vi "ADstar on a Dynamic Occupancy Grid - Copy.vi"() -> ()   [LabVIEW 2012]
doc: "This example continually replans a path from Start to Goal while following the best known path, including through obstacles if necessary.\nThe Anytime D* search algorithm is useful when the world or the robot's understanding of the world is changing. Anytime D* maintains more information than the A* search algorithm so the robot can backtrack and find a new path more easily if it discovers the original path will not work."
uses:
  <vilib>/robotics/Navigation/shared/WorldMap/OccupancyGridWorldMap/NI_Robotics_OccupancyGridWorldMap.lvclass
  <vilib>/robotics/Navigation/Anytime D Star/NI_Robotics_AnytimeDStar.lvclass
panel:
  in  "Step Through":bool
  in  "goal y":i32=49
  in  "goal x":i32=49
  out "Open List Size":i32(graph)=1665
  out "path on obstacles":dbl[][](graph)
  out "AD* Open Nodes":i32=1665 caption="size"
  out "Path Cost":dbl(graph)
  in  "Epsilon":i32=2 min=1
  out "AD* Path Cost":dbl caption="path cost"
  in  "y start":i32
  in  "x start":i32
  in  "Move Robot":i32=1 min=0
  in  "Overhaul":i32=25
  in  "step button":bool
  out "AD* Time":u32=117 caption="seconds"
  out "Compute Path Time":u32(graph)=117
  in  "stop":bool
  # "The Anytime D* search algorithm is useful when the world or the robot's understanding of the world is changing.  Anytime D* maintains more information\n than the A* search algorithm so the robot can backtrack and find a new path more easily if it discovers the original path will not work."
  # "This example continually replans a path from Start to Goal while \nfollowing the best known path, including through obstacles if necessary."
  # "Configuration"
  # "X"
  # "Y"
  # "Start"
  # "Goal"
  # "Run Mode"
  # "Run-time Control"
  # "Detection radius of robot's sensors."
  # "Number of steps the robot takes after each plan."
  # "Number of steps before AD* plans from scratch."
  # "1) Choose the Start and Goal location and the % Random Obstacles.\n2) Run the VI.\n3) Adjust the controls in the Run-time Controls section to see the \n     effect each option has on path planning\n4) Change the Run Mode to Single Step to pause after each time\n the AD* VI runs"
  # "A higher epsilon results in a faster but less optimal search."
  # "Continuous"
  # "Single Step"
  # "Robot"
  # "Obstacle"
  # "Unknown"
  # "Free"
  # "Path"
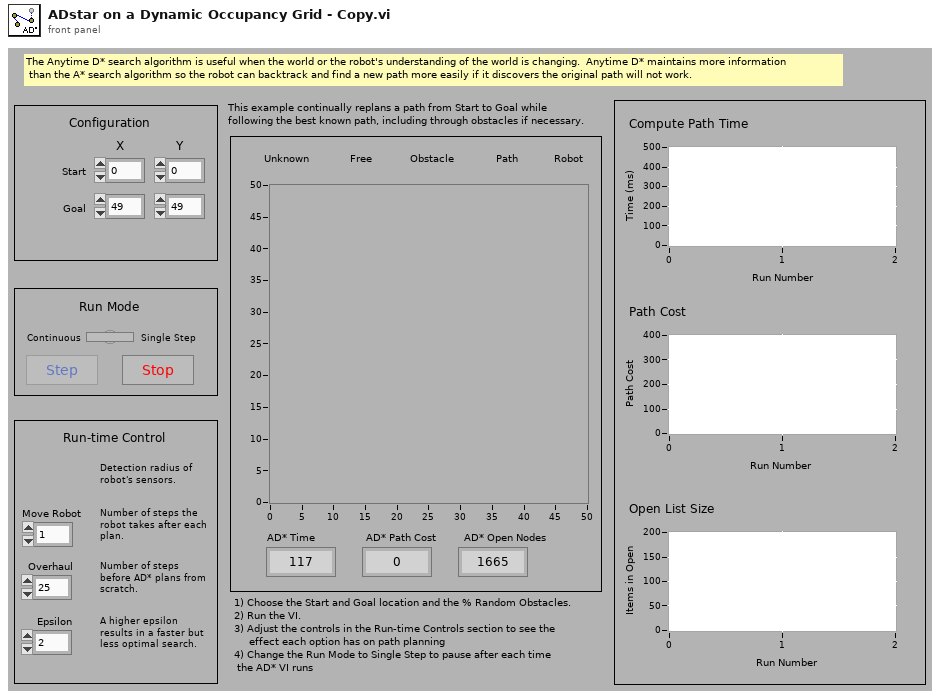
[diagram p1: front panel]
types:
  T1 = enum8{"Enabled", "Disabled", "Disabled and Grayed Out"}
  T2 = cluster{"epsilon":dbl, "run number":i32, "open list size":i32}
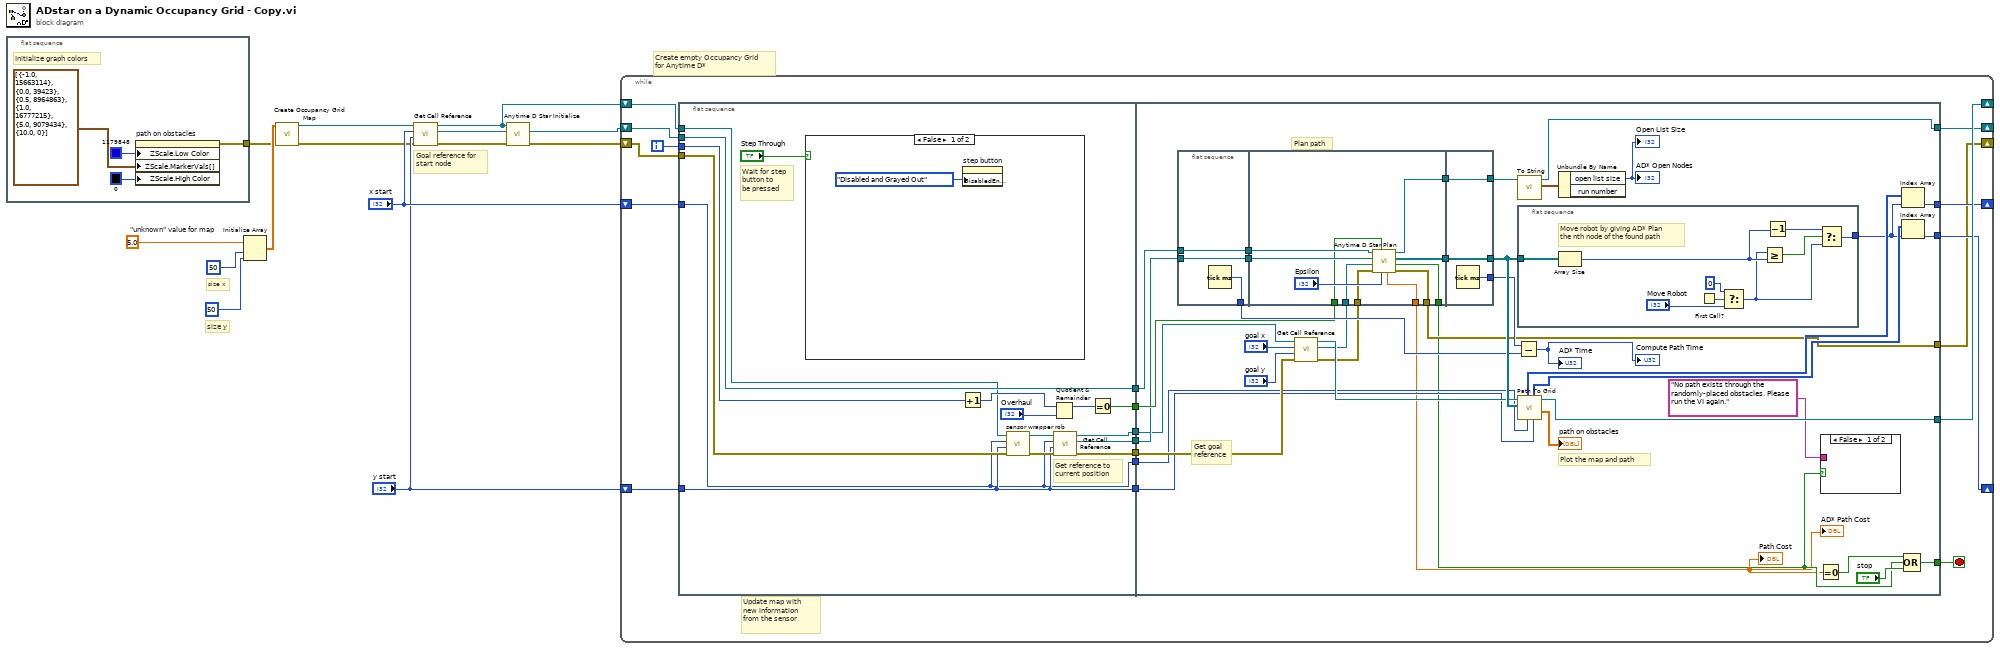
[diagram p0: block diagram]
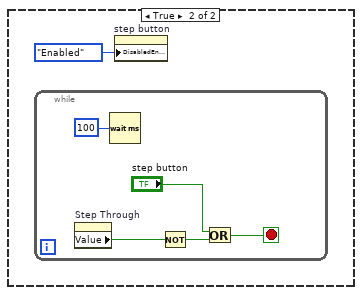
[diagram p2: hidden frame]
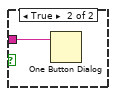
[diagram p3: hidden frame]
diagram:
  w12 = 5.0  # "unknown" value for map
  # "Goal reference for\nstart node"
  # "size y"
  # "size x"
  # "Create empty Occupancy Grid\nfor Anytime D*"
  n1 = flat-sequence {
    tunnel: [w15] -> w5
    frame #0 {
      # "Initialize graph colors"
      n2 = property on="path on obstacles" class="IntGraph (strict)"("ZScale.Low Color"=u32 1179848, "ZScale.MarkerVals[]"=cluster{dbl, u32}[] [{-1.0, 15663114}, {0.0, 39423}, {0.5, 8964863}, {1.0, 16777215}, {5.0, 9079434}, {10.0, 0}], "ZScale.High Color"=u32 0) -> (error out=w15:errorcluster)  [unwired: 2 in, 1 out]
    }
  }
  n3 = Initialize Array(w12, 50 ("y"), 50 ("x")) -> (w9:dbl[][])
  n4 = call <vilib>:"Create Occupancy Grid Map.vi"("error in (no error)"=w5, "occupancy grid"=w9) -> ("error out"=w7:errorcluster, "map reference out"=w2:refnum<data-value>)  [unwired: 8 in]
  n5 = call <vilib>:"Get Cell Reference.vi"("error in (no error)"=w7, "y"="y start", "x"="x start", "map reference in"=w2) -> ("error out"=w6:errorcluster, "cell reference"=w8:refnum<data-value>, "map reference out"=w3:refnum<data-value>)  [unwired: 4 in, 1 out]
  n6 = call <vilib>:"Anytime D Star Initialize.vi"("error in (no error)"=w6, "start reference"=w8, "map reference in"=w3) -> ("error out"=w1:errorcluster, "Anytime D*"=w4:refnum<class "NI_Robotics_AnytimeDStar.lvclass">)  [unwired: 7 in]
  n7 = while {
    shift-right: [w32] -> _
    shift-left: w4 -> [w37]
    shift-right: [w36] -> _
    shift-left: w3 -> [w22]
    shift-right: [w31] -> _
    shift-left: "x start" -> [w19]
    shift-right: [w30] -> _
    shift-left: "y start" -> [w20]
    shift-right: [w26] -> _
    shift-left: w1 -> [w21]
    i -> [w29]
    stop <- w23 stop-if-true
    # "Update map with new information\nfrom the sensor"
    n8 = flat-sequence {
      tunnel: w29 -> [w46]
      tunnel: w22 -> [w43]
      tunnel: w37 -> [w53]
      tunnel: [w53] -> w35
      tunnel: [w52] -> w34
      tunnel: [w51] -> w33
      tunnel: w19 -> [w38]
      tunnel: w20 -> [w39]
      tunnel: [w45] -> w28
      tunnel: w21 -> [w40]
      tunnel: [w44] -> w27
      tunnel: [w38] -> w25
      tunnel: [w39] -> w24
      tunnel: [w63] -> w23
      tunnel: [w97] -> w32
      tunnel: [w85] -> w36
      tunnel: [w78] -> w31
      tunnel: [w77] -> w30
      tunnel: w28 -> [w83]
      tunnel: w33 -> [w82]
      tunnel: w34 -> [w76]
      tunnel: w35 -> [w93]
      tunnel: w27 -> [w73]
      tunnel: [w69] -> w26
      tunnel: w25 -> [w68]
      tunnel: w24 -> [w67]
      frame #0 {
        # "Get reference to \ncurrent position"
        # "Wait for step\nbutton to\nbe pressed"
        n9 = case shown="False" "Step Through" {
          frame False {
            n10 = property on="step button" class="Bool"("DisabledEnum"=T1."Disabled and Grayed Out" ("Disabled")) -> ()  [unwired: 2 in, 2 out]
          }
          frame True {
            n11 = while {
              stop <- w58 stop-if-true
              n12 = property on="Step Through" class="Bool (strict)"() -> ("Value"=w56:bool)  [unwired: 2 in, 2 out]
              n13 = Wait (ms)(milliseconds to wait=u32 100) -> ()  [unwired: 1 out]
              n14 = Not(x=w56) -> (.not. x?=w57:bool)
              n15 = Or(x="step button", y=w57) -> (x .or. y?=w58:bool)
            }
            n16 = property on="step button" class="Bool"("DisabledEnum"=T1."Enabled" ("Disabled")) -> ()  [unwired: 2 in, 2 out]
          }
        }
        n17 = Increment(x=w46) -> (x+1=w48:i32)
        n18 = call "sensor wrapper rob.vi"("error in (no error)"=w40, "sensor y"=w39, "Sensor x"=w38, "map reference in"=w43) -> ("error out"=w41:errorcluster, "map reference out 2"=w42:refnum<data-value>)  [unwired: 6 in]
        n19 = Quotient & Remainder(x=w48, y="Overhaul") -> (x-y*floor(x/y)=w47:i32)  [unwired: 1 out]
        n20 = call <vilib>:"Get Cell Reference.vi"("error in (no error)"=w41, "y"=w39, "x"=w38, "map reference in"=w42) -> ("error out"=w44:errorcluster, "cell reference"=w51:refnum<data-value>, "map reference out"=w52:refnum<data-value>)  [unwired: 4 in, 1 out]
        n21 = Equal To 0?(x=w47) -> (x = 0?=w45:bool)
      }
      frame #1 {
        # "Plot the map and path"
        # "Get goal \nreference"
        # "Plan path"
        n22 = flat-sequence {
          tunnel: w93 -> [w110]
          tunnel: w82 -> [w111]
          tunnel: [w111] -> w92
          tunnel: [w110] -> w91
          tunnel: [w109] -> w87
          tunnel: [w118] -> w64
          tunnel: [w117] -> w62
          tunnel: w92 -> [w121]
          tunnel: w91 -> [w122]
          tunnel: [w119] -> w90
          tunnel: [w120] -> w89
          tunnel: w83 -> [w115]
          tunnel: w71 -> [w114]
          tunnel: w70 -> [w113]
          tunnel: [w112] -> w69
          tunnel: [w124] -> w96
          tunnel: [w125] -> w98
          tunnel: w90 -> [w125]
          tunnel: w89 -> [w124]
          tunnel: [w123] -> w88
          frame #0 {
            n23 = Tick Count (ms)() -> (millisecond timer value=w109:u32)
          }
          frame #1 {
            n24 = call <vilib>:"Anytime D Star Plan.vi"("epsilon"="Epsilon", "overhaul (F)"=w115, "error in (no error)"=w113, "new goal reference"=w114, "current reference"=w121, "Anytime D* in"=w122) -> ("error out"=w112:errorcluster, "no valid path exists"=w118:bool, "path references"=w120:refnum<data-value>[], "Anytime D* out"=w119:refnum<class "NI_Robotics_AnytimeDStar.lvclass">, "path cost"=w117:dbl)  [unwired: 1 in]
          }
          frame #2 {
            n25 = Tick Count (ms)() -> (millisecond timer value=w123:u32)
          }
        }
        n26 = call <vilib>:"Get Cell Reference.vi"("error in (no error)"=w73, "y"="goal y", "x"="goal x", "map reference in"=w76) -> ("error out"=w70:errorcluster, "cell reference"=w71:refnum<data-value>, "map reference out"=w72:refnum<data-value>)  [unwired: 4 in, 1 out]
        n27 = Subtract(x=w88, y=w87) -> (x-y=→"Compute Path Time" →"AD* Time":u32)
        n28 = call <vilib>:"To String.vi"("Anytime D* in"=w98) -> ("output"=w95:T2, "Anytime D* out"=w97:refnum<class "NI_Robotics_AnytimeDStar.lvclass">)  [unwired: 8 in, 1 out]
        n29 = flat-sequence {
          tunnel: w96 -> [w107]
          tunnel: [w100] -> w79
          frame #0 {
            # "Move robot by giving AD* Plan\nthe nth node of the found path"
            n30 = Array Size(array=w107) -> (size(s)=w104:i32)
            n31 = First Call?() -> (First Call?: T/F=w106:bool)
            n32 = Select(t=0, s=w106, f="Move Robot") -> (s? t:f=w103:i32)
            n33 = Greater Or Equal?(x=w103, y=w104) -> (x >= y?=w102:bool)
            n34 = Decrement(x=w104) -> (x-1=w108:i32)
            n35 = Select(t=w108, s=w102, f=w103) -> (s? t:f=w100:i32)
          }
        }
        n36 = call "Path To Grid.vi"("current y"=w67, "current x"=w68, "path references"=w96, "map reference in"=w72) -> ("path on obstacles"=→"path on obstacles":dbl[][], "map reference out"=w85:refnum<data-value>, "y coordinates"=w81:i32[], "x coordinates"=w80:i32[])  [unwired: 3 in, 1 out]
        n37 = Unbundle By Name(w95) -> ("open list size"=→"Open List Size" →"AD* Open Nodes":i32)  [unwired: 1 out]
        n38 = Equal To 0?(x=w62) -> (x = 0?=w61:bool)
        n39 = case shown="False" w64 {
          tunnel: "No path exists through the randomly-placed obstacles. Please run the VI again." -> [_ w99]
          frame False {
          }
          frame True {
            n40 = One Button Dialog(message=w99) -> ()  [unwired: 1 in, 1 out]
          }
        }
        n41 = Index Array(array=w80, index=w79) -> (element=w78:i32)
        n42 = Index Array(array=w81, index=w79) -> (element=w77:i32)
        n43 = Compound Arithmetic op=OR(w61, w64, "stop") -> (w63:bool)
        "AD* Path Cost" <- w62
        "Path Cost" <- w62
      }
    }
  }
